vi "Path_2_String.vi"(1 "POSIXFormattedPseudopath (F)":bool, 2 "Real Path":path) -> (0 "Path String":string)   [LabVIEW 2015]
uses:
  Globals/Constants_global.vi
panel:
  out "Data Folder":path
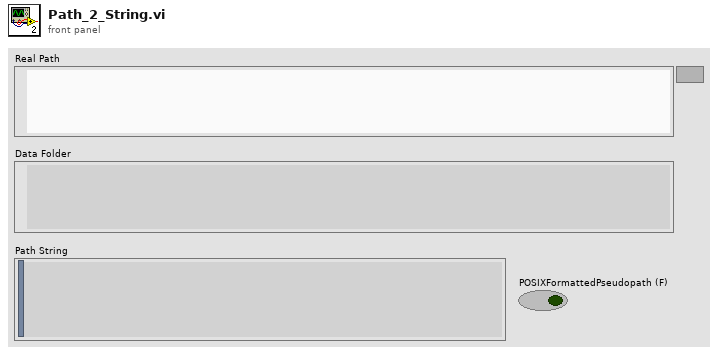
[diagram p1: front panel]
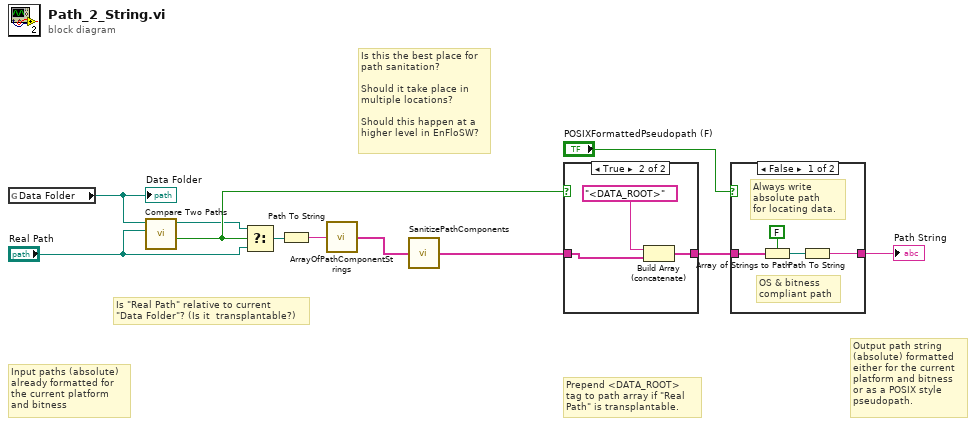
[diagram p0: block diagram]
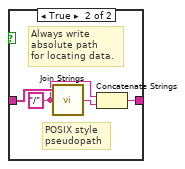
[diagram p2: hidden frame]
diagram:
  # "Is this the best place for\npath sanitation?\n\nShould it take place in\nmultiple locations?\n\nShould this happen at a\nhigher level in EnFloSW?"
  # "Input paths (absolute)\nalready formatted for\nthe current platform \nand bitness"
  # "Is \"Real Path\" relative to current\n\"Data Folder\"? (Is it  transplantable?)"
  # "Prepend <DATA_ROOT>\ntag to path array if \"Real\nPath\" is transplantable."
  # "Input paths (absolute)\nalready formatted for\nthe current platform \nand bitness"
  # "Output path string\n(absolute) formatted\neither for the current\nplatform and bitness\nor as a POSIX style\npseudopath."
  n1 = global read "Constants_global.vi" "Data Folder"() -> (w11:path)
  "Data Folder" <- w11
  n2 = call <vilib>:"Compare Two Paths.vi"("Path 2"="Real Path", "Path 1"=w11) -> ("Path 2 Relative to Path 1?"=w10:bool, "Relative Path from 1 to 2"=w8:path)  [unwired: 6 in, 2 out]
  n3 = Select(t=w8, s=w10, f="Real Path") -> (s? t:f=w7:path)
  n4 = Path To String(path=w7) -> (string=w3:string)
  n5 = call "ArrayOfPathComponentStrings.vi"("PathStringIn"=w3) -> ("ArrayOfPathComponentStringsOut"=w1:string[])
  n6 = call "SanitizePathComponents.vi"("PathComponentsIn"=w1) -> ("SanitizedComponentsOut"=w2:string[])
  n7 = case shown="True" w10 {
    tunnel: [w12 w14] -> w6
    tunnel: w2 -> [w12 w13]
    frame False {
    }
    frame True {
      n8 = Build Array (concatenate)("<DATA_ROOT>", w13) -> (w14:string[])
    }
  }
  n9 = case shown="False" "POSIXFormattedPseudopath (F)" {
    tunnel: w6 -> [w16 w23]
    tunnel: [w17 w22] -> w5
    frame False {
      # "OS & bitness\ncompliant path"
      # "Always write\nabsolute path\nfor locating data."
      n10 = Array of Strings to Path(0:w16, 1:FALSE ("relative")) -> (2:w18:path)
      n11 = Path To String(path=w18) -> (string=w17:string)
    }
    frame True {
      w20 = "/" ("Separator (,)")
      # "POSIX style\npseudopath"
      # "Always write\nabsolute path\nfor locating data."
      n12 = call <vilib>:"Join Strings.vi"("Separator (,)"=w20, "Strings In"=w23) -> ("String"=w21:string)  [unwired: 1 in]
      n13 = Concatenate Strings(w20, w21) -> (w22:string)
    }
  }
  "Path String" <- w5
